vi "Write Cursor Params.vi"(8 "error in (no error)":errorcluster, 10 "output cluster":T1, 11 "MassSpectrumExtractor in":refnum<class "MassSpectrumExtractor.lvclass">) -> (0 "error out":errorcluster, 3 "MassSpectrumExtractor out":refnum<class "MassSpectrumExtractor.lvclass">)   [LabVIEW 2014]
uses:
  MassSpectrumExtractor.lvclass
  Cursor params.ctl
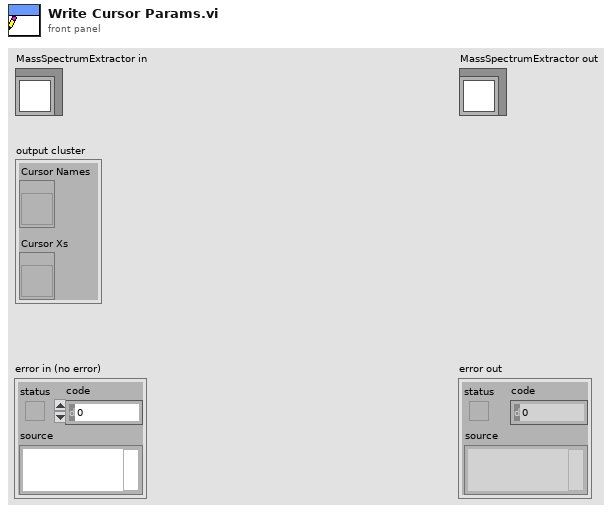
[diagram p1: front panel]
types:
  T1 = typedef "MassSpectrumExtractor.lvclass/Cursor params.ctl" = cluster{"Cursor Xs":refnum<vi>, "Cursor Names":refnum<vi>}
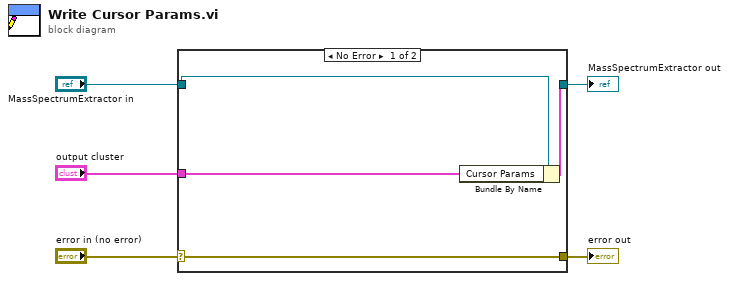
[diagram p0: block diagram]
diagram:
  n1 = case shown="No Error" "error in (no error)" {
    selector: "error in (no error)" -> [w9 w10]
    tunnel: [w9 w10] -> w4
    tunnel: [w7 w11] -> w2
    tunnel: "MassSpectrumExtractor in" -> [w8 w11]
    tunnel: "output cluster" -> [w6 _]
    frame No Error {
      n2 = Bundle By Name(cluster=w8, "Cursor Params"=w6) -> (w7:cluster{})
    }
    frame Error {
    }
  }
  "error out" <- w4
  "MassSpectrumExtractor out" <- w2
